vi "Find missing TDMS files.vi"() -> ()   [LabVIEW 2016, in "Retrieve and Visualize.lvclass"]
uses:
  Retrieve and Visualize.lvclass
  <userlib>/LevyLab/LV-Data/LV-Data/Typedefs/File Type--enum.ctl
  <userlib>/LevyLab/LV-Data/LV-Data/LV-Data.lvclass
panel:
  in  "Trial Run":bool
  out "Missing FIiless":path[](array[path])
  out "found number?":bool
  out "slow*fast":i32
  out "slow*fast = number?":bool
  in  "fast":i32
  in  "slow":i32
  out "number of missing files":i32
  out "number of files":i32
  in  "Folder Path":path
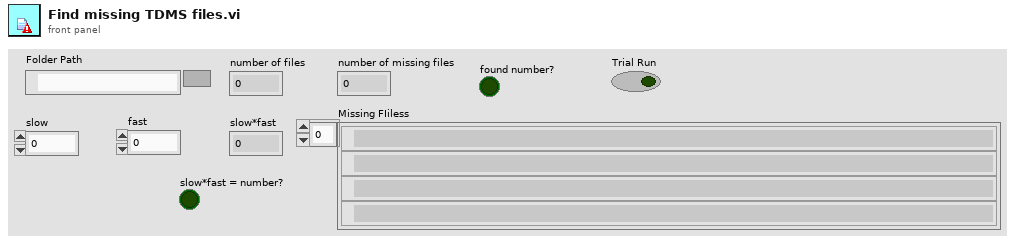
[diagram p1: front panel]
types:
  T1 = typedef "LV-Data.lvclass/File Type--enum.ctl" = enum16{"DAT", "ITX", "TDMS", "VI"}
  T2 = typedef "LV-Data.lvclass/Dictionary--cluster.ctl" = cluster{"key":string, "value":variant}
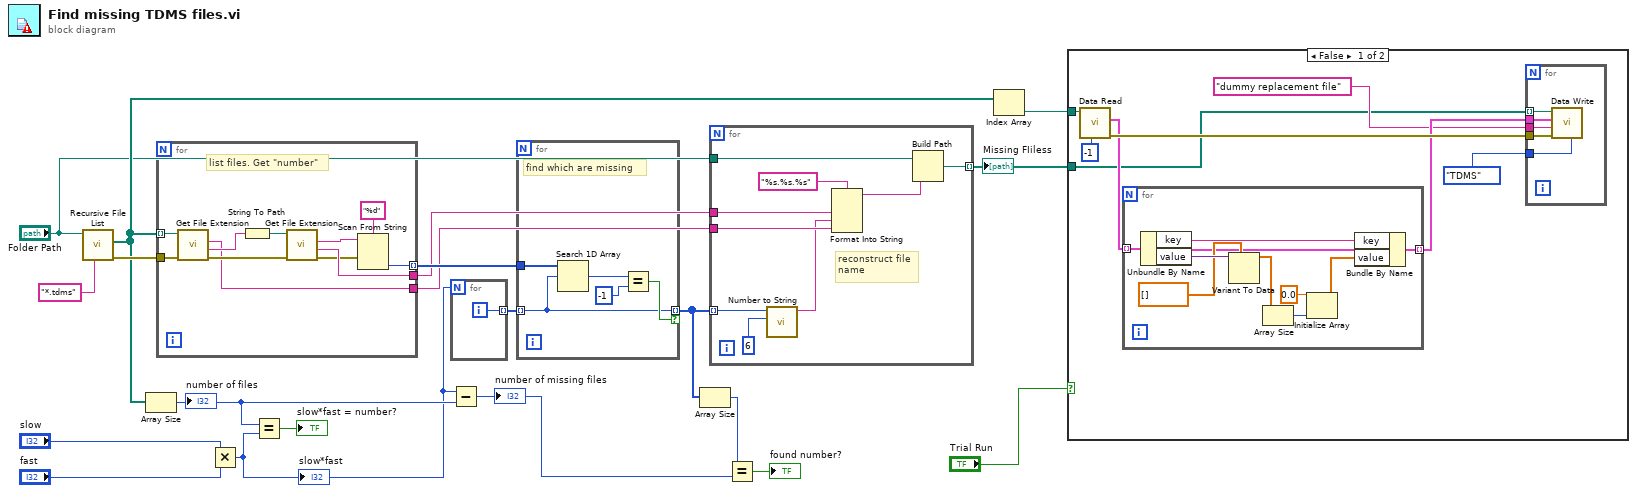
[diagram p0: block diagram]
diagram:
  n1 = call <vilib>:"Recursive File List.vi"("pattern"="*.tdms", "Folder Path"="Folder Path") -> ("error out"=w19:errorcluster, "All Files in Dir"=w5:path[])  [unwired: 5 in, 3 out]
  n2 = Array Size(array=w5) -> (size(s)=w16:i32)
  "number of files" <- w16
  n3 = for {
    tunnel: w5 -> [w25] mode=indexing
    tunnel: w19 -> [w31]
    tunnel: [w26] -> w18 mode=indexing
    tunnel: [w24] -> w11
    tunnel: [w21] -> w10
    # "list files. Get \"number\""
    n4 = call <vilib>:"Get File Extension.vi"("error in (no error)"=w31, "file"=w25) -> ("error out"=w29:errorcluster, "filename without extension"=w28:string, "lowercase file extension"=w21:string)  [unwired: 5 in, 2 out]
    n5 = String To Path(string=w28) -> (path=w30:path)
    n6 = call <vilib>:"Get File Extension.vi"("error in (no error)"=w29, "file"=w30) -> ("error out"=w22:errorcluster, "filename without extension"=w24:string, "lowercase file extension"=w23:string)  [unwired: 5 in, 2 out]
    n7 = Scan From String(format string="%d", input string=w23, error in=w22) -> (output 1=w26:i32)  [unwired: 2 in, 3 out]
  }
  n8 = Multiply(x="slow", y="fast") -> (x*y=w12:i32)
  "slow*fast" <- w12
  n9 = Equal?(x=w16, y=w12) -> (x = y?=→"slow*fast = number?":bool)
  n10 = for {
    N: w12 -> [_]
    tunnel: [w32] -> w17 mode=indexing
    i -> [w32]
  }
  n11 = Subtract(x=w12, y=w16) -> (x-y=w8:i32)
  "number of missing files" <- w8
  n12 = for {
    tunnel: [w34] -> w6 mode=indexing if=w36
    tunnel: w18 -> [w35]
    tunnel: w17 -> [w34] mode=indexing
    # "find which are missing"
    n13 = Search 1D Array(1D array=w35, element=w34) -> (index of element=w33:i32)  [unwired: 1 in]
    n14 = Equal?(x=w33, y=-1) -> (x = y?=w36:bool)
  }
  n15 = Array Size(array=w6) -> (size(s)=w9:i32)
  n16 = for {
    tunnel: w6 -> [w45] mode=indexing
    tunnel: w11 -> [w43]
    tunnel: w10 -> [w42]
    tunnel: [w38] -> w2 mode=indexing
    tunnel: "Folder Path" -> [w40]
    # "reconstruct file\nname"
    n17 = call <userlib>:"Number to String.vi"("desired minimum string length"=6, "Number"=w45) -> ("String"=w41:string)  [unwired: 8 in, 1 out]
    n18 = Format Into String(format string="%s.%s.%s", w43, w41, w42) -> (resulting string=w39:string)  [unwired: 2 in, 1 out]
    n19 = Build Path(base path=w40, name or relative path=w39) -> (appended path=w38:path)
  }
  "Missing FIiless" <- w2
  n20 = Equal?(x=w9, y=w8) -> (x = y?=→"found number?":bool)
  n21 = Index Array(array=w5) -> (element=w4:path)  [unwired: 1 in]
  n22 = case shown="False" "Trial Run" {
    tunnel: w4 -> [w54 _]
    tunnel: w2 -> [w47 _]
    frame False {
      n23 = call <userlib>:"Data Read.vi"("Append Index"=-1, "path"=w54) -> ("error out"=w52:errorcluster, "Data (Dictionary)"=w51:T2[])  [unwired: 6 in, 2 out]
      n24 = for {
        tunnel: w51 -> [w63] mode=indexing
        tunnel: [w60] -> w50 mode=indexing
        n25 = Unbundle By Name(w63) -> ("key"=w62:string, "value"=w68:variant)
        n26 = Variant To Data(type=dbl[] [], Variant=w68) -> (data=w66:dbl[])  [unwired: 1 in, 1 out]
        n27 = Array Size(array=w66) -> (size(s)=w65:i32)
        n28 = Initialize Array(0.0 ("element"), w65) -> (w61:dbl[])
        n29 = Bundle By Name(cluster=w63, "key"=w62, "value"=w61) -> (w60:T2)
      }
      n30 = for {
        tunnel: w52 -> [w59]
        tunnel: w50 -> [w58]
        tunnel: File_Type--enum."TDMS" ("File Type") -> [w57]
        tunnel: "dummy replacement file" ("Notes") -> [w56]
        tunnel: w47 -> [w55] mode=indexing
        n31 = call <userlib>:"Data Write.vi"("File Type"=w57, "error in (no error)"=w59, "Notes"=w56, "Data (Dictionary)"=w58, "path"=w55) -> ()  [unwired: 5 in, 2 out]
      }
    }
    frame True {
    }
  }
